vi "LV2G_Mono_GratLookup.vi"(7 "Operation":T1, 8 "error in (no error)":errorcluster, 11 "lookup":string[][](array[string])) -> (0 "error out":errorcluster, 2 "lookupOut1":dbl[][](array[numeric]), 3 "lookupOut":string[][](array[string]))   [LabVIEW 2018]
uses:
  Strict Type Controls/Settings Operation.ctl
  <vilib>/Utility/file.llb/Read From Spreadsheet File (string).vi
  <vilib>/Utility/file.llb/Write To Spreadsheet File (string).vi
panel:
  # "N1\t93,81\nN2\t157,81\nN3\t92,114\nN4\t157,80"
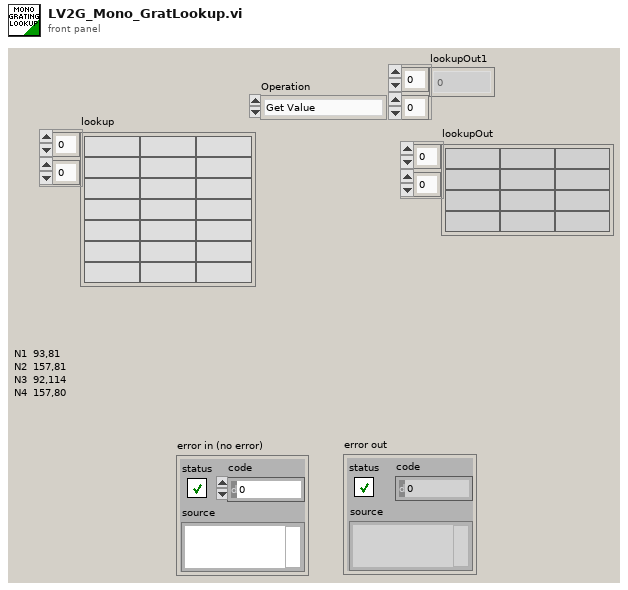
[diagram p1: front panel]
types:
  T1 = typedef "Settings Operation.ctl" = enum8{"Get Value", "Set Value", "Read File", "Write File", "Write Stored Value"}
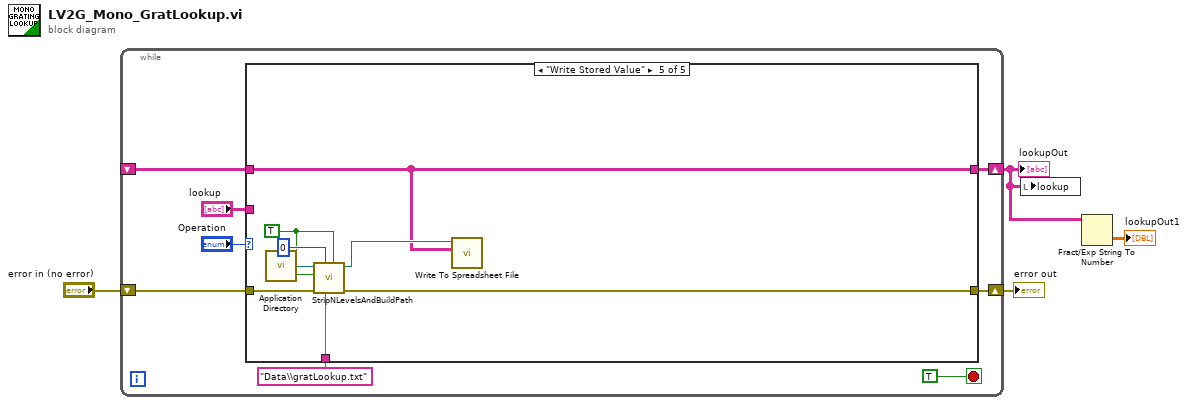
[diagram p0: block diagram]
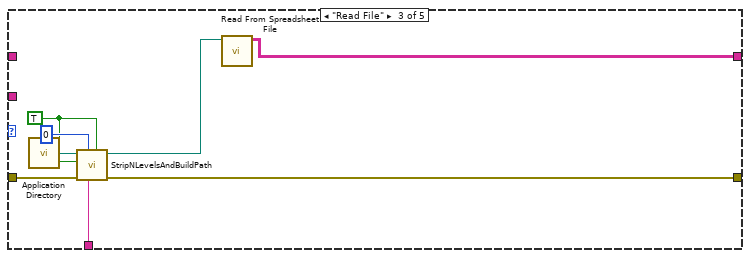
[diagram p4: hidden frame]
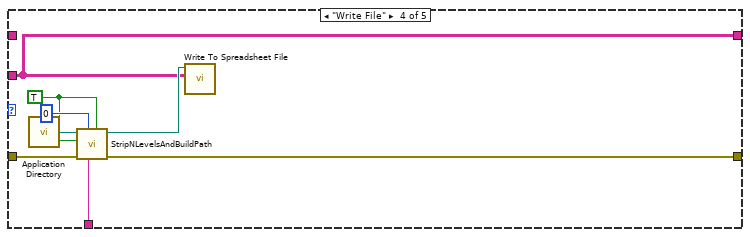
[diagram p5: hidden frame]
diagram:
  n1 = while {
    shift-right: [w11] -> w2
    shift-left: _ -> [w12]
    shift-right: [w8] -> w3
    shift-left: "error in (no error)" -> [w9]
    stop <- TRUE stop-if-true
    n2 = case shown="\"Write Stored Value\"" "Operation" {
      tunnel: w12 -> [w14 _ _ _ w34]
      tunnel: [w14 w16 w18 w26 w34] -> w11
      tunnel: "lookup" -> [_ w16 _ w26 _]
      tunnel: w9 -> [w13 w15 w21 w31 w37]
      tunnel: [w13 w15 w17 w25 w33] -> w8
      tunnel: "Data\\gratLookup.txt" ("Build Path") -> [_ _ w20 w28 w36]
      frame "Get Value" {
      }
      frame "Set Value" {
      }
      frame "Read File" {
        w22 = TRUE ("Is File?")
        n3 = call <vilib>:"Application Directory.vi"() -> ("Application Directory"=w24:path)
        n4 = call "StripNLevelsAndBuildPath.vi"("Create Folders"=w22, "Build Path"=w20, "Strip Levels"=0, "error in(no error)"=w21, "Is File"=w22, "Path In"=w24) -> ("error out"=w17:errorcluster, "Path Out"=w19:path)  [unwired: 4 out]
        n5 = call-poly <vilib>:"Read From Spreadsheet File.vi"("file path (dialog if empty)"=w19) -> ("all rows"=w18:string[][])  [unwired: 6 in, 4 out]
      }
      frame "Write File" {
        w29 = TRUE ("Is File?")
        n6 = call <vilib>:"Application Directory.vi"() -> ("Application Directory"=w32:path)
        n7 = call "StripNLevelsAndBuildPath.vi"("Create Folders"=w29, "Build Path"=w28, "Strip Levels"=0, "error in(no error)"=w31, "Is File"=w29, "Path In"=w32) -> ("error out"=w25:errorcluster, "Path Out"=w27:path)  [unwired: 4 out]
        n8 = call-poly <vilib>:"Write To Spreadsheet File.vi"("2D data"=w26, "file path (dialog if empty)"=w27) -> ()  [unwired: 6 in, 1 out]
      }
      frame "Write Stored Value" {
        w38 = TRUE ("Is File?")
        n9 = call <vilib>:"Application Directory.vi"() -> ("Application Directory"=w40:path)
        n10 = call "StripNLevelsAndBuildPath.vi"("Create Folders"=w38, "Build Path"=w36, "Strip Levels"=0, "error in(no error)"=w37, "Is File"=w38, "Path In"=w40) -> ("error out"=w33:errorcluster, "Path Out"=w35:path)  [unwired: 4 out]
        n11 = call-poly <vilib>:"Write To Spreadsheet File.vi"("2D data"=w34, "file path (dialog if empty)"=w35) -> ()  [unwired: 6 in, 1 out]
      }
    }
  }
  "error out" <- w3
  "lookupOut" <- w2
  n12 = local write "lookup"(w2) -> ()
  n13 = Fract/Exp String To Number(string=w2) -> (number=→"lookupOut1":dbl[][])  [unwired: 3 in, 1 out]
